vi "lv_mysql_conn_receive_data_packet.vi"(8 "error in":errorcluster, 9 "timeout ms (5000)":i32=5000, 11 "connection ID":refnum<k5>) -> (0 "error out":errorcluster, 1 "TCP/IP Data":u8[](array[numeric]), 2 "Packet #":u8, 3 "connection ID out":refnum<k5>)   [LabVIEW 2015]
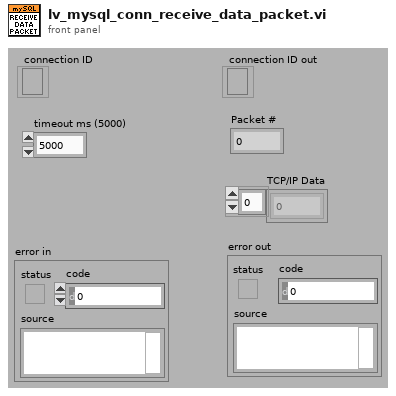
[diagram p1: front panel]
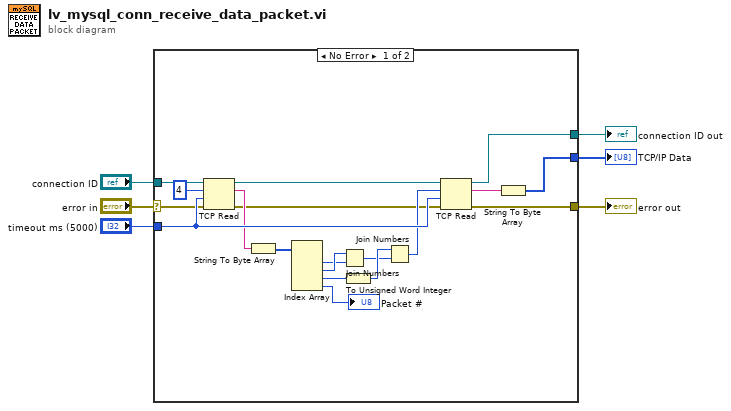
[diagram p0: block diagram]
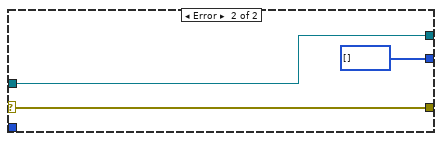
[diagram p2: hidden frame]
diagram:
  n1 = case shown="No Error" "error in" {
    selector: "error in" -> [w10 w26]
    tunnel: [w25 w27] -> w6
    tunnel: "timeout ms (5000)" -> [w23 _]
    tunnel: "connection ID" -> [w12 w27]
    tunnel: [w8 w26] -> w3
    tunnel: [w9 u8[] [] ("unsigned byte array")] -> w2
    frame No Error {
      n2 = TCP Read(connection ID=w12, bytes to read=4, error in (no error)=w10, 9:w23) -> (connection ID out=w7:refnum<k5>, data out=w15:string, error out=w14:errorcluster)  [unwired: 1 in]
      n3 = String To Byte Array(string=w15) -> (unsigned byte array=w16:u8[])
      n4 = Index Array(array=w16) -> (element #1=w17:u8, element #2=w18:u8, element #3=w21:u8, element #4=→"Packet #":u8)  [unwired: 4 in]
      n5 = Join Numbers(hi=w18, lo=w17) -> ((hi.lo)=w19:u16)
      n6 = To Unsigned Word Integer(number=w21) -> (unsigned 16bit integer=w20:u16)
      n7 = Join Numbers(hi=w20, lo=w19) -> ((hi.lo)=w22:u32)
      n8 = TCP Read(connection ID=w7, bytes to read=w22, error in (no error)=w14, 9:w23) -> (connection ID out=w25:refnum<k5>, data out=w11:string, error out=w8:errorcluster)  [unwired: 1 in]
      n9 = String To Byte Array(string=w11) -> (unsigned byte array=w9:u8[])
    }
    frame Error {
    }
  }
  "connection ID out" <- w6
  "error out" <- w3
  "TCP/IP Data" <- w2
